vi "ASYNC_Adam_client.vi"(2 "Values":dbl[](array[numeric]) format="%.2f", 3 "Check Value is in the scan table?":bool, 4 "Channel Names":string[](array[string])) -> (0 "Scan Comments":string[](array[string]), 1 "Calibrated Units":dbl[](array[numeric]) format="%.4f")   [LabVIEW 2017]
uses:
  Anemometry/Anemometry Sub Vis/Controls/Global_mode.ctl
  Sub VIs/ADAM Controls/Update_scan_value.ctl
  Anemometry/Anemometry Sub Vis/Globals/Preference_global.vi
panel:
  out "Iterations":i32
  in  "ASYNC Adam server":refnum<vi>
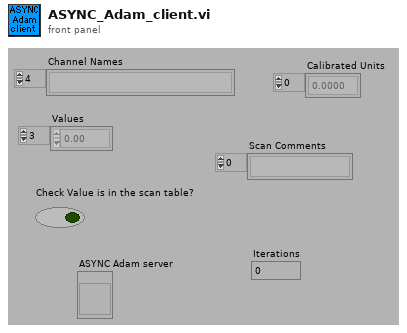
[diagram p1: front panel]
types:
  T1 = typedef "Server_Comms.ctl" = enum16{"Server Link Healthy", "Do Not Link To Server"}
  T2 = typedef "Update_scan_value.ctl" = cluster{"Channel Name":string, "New Value":dbl}
  T3 = typedef "Global_mode.ctl" = enum16{"Read Global", "Load Global From File", "Write Global to File"}
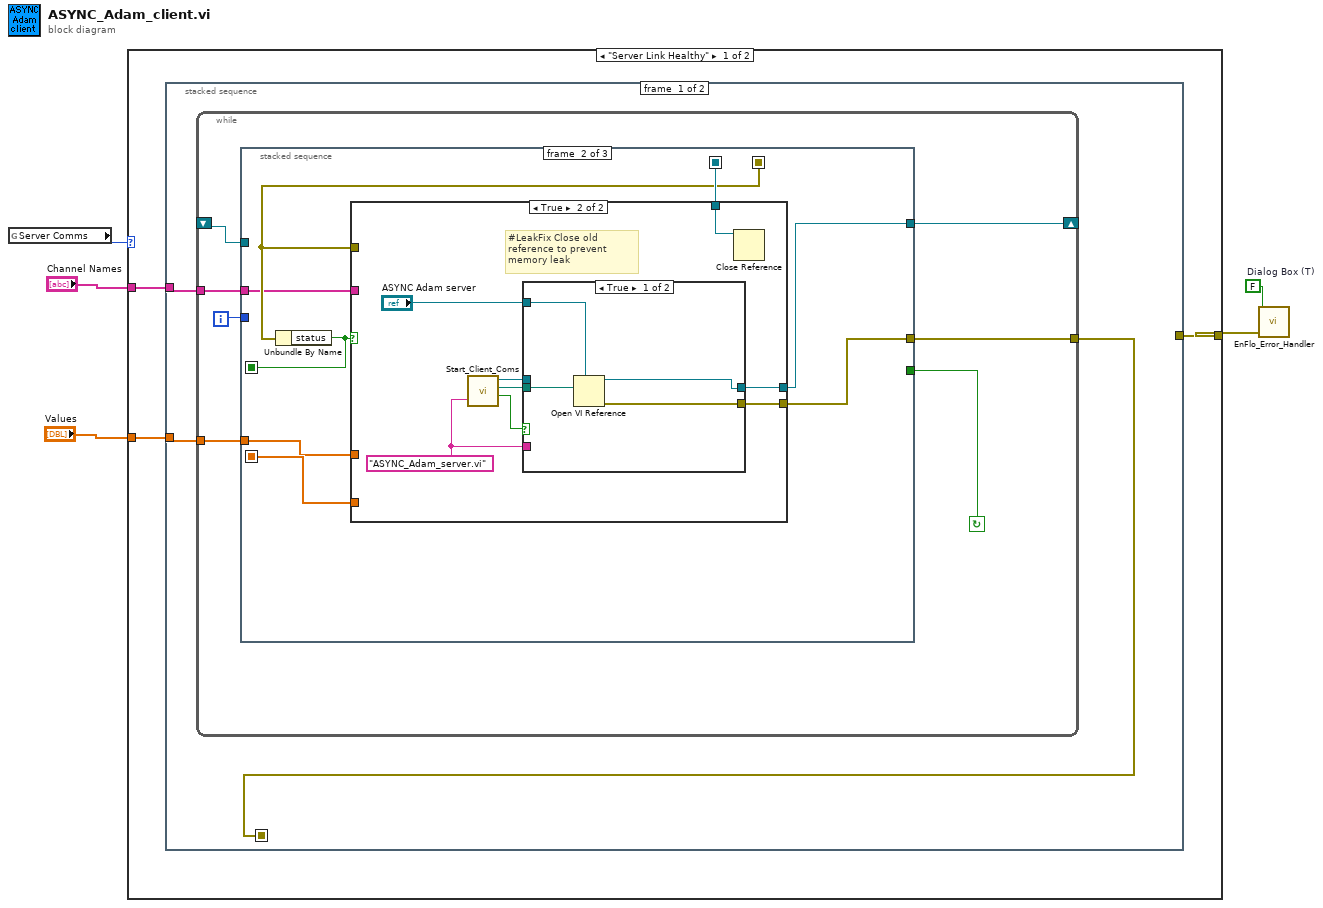
[diagram p0: block diagram]
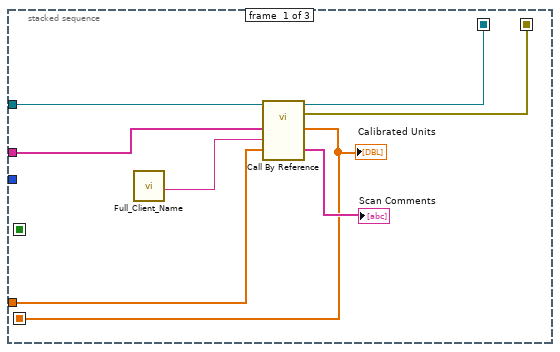
[diagram p2: hidden frame]
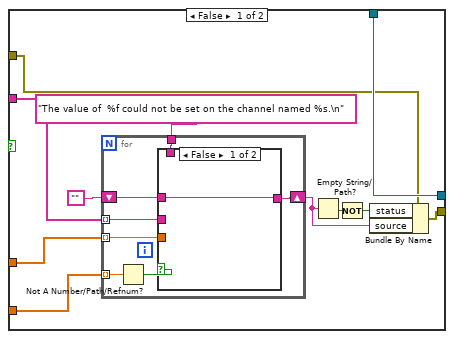
[diagram p3: hidden frame]
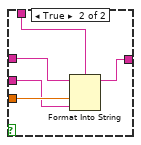
[diagram p4: hidden frame]
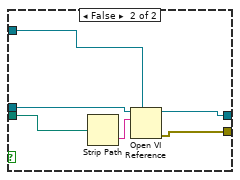
[diagram p5: hidden frame]
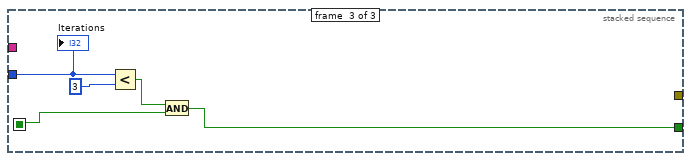
[diagram p6: hidden frame]
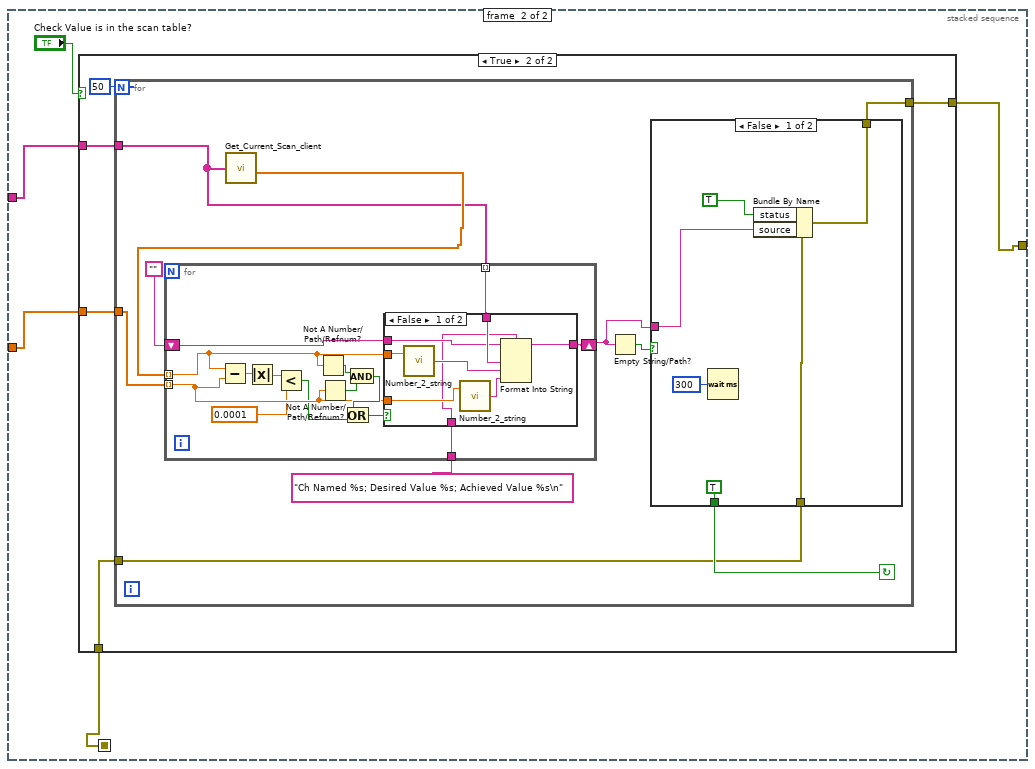
[diagram p7: hidden frame]
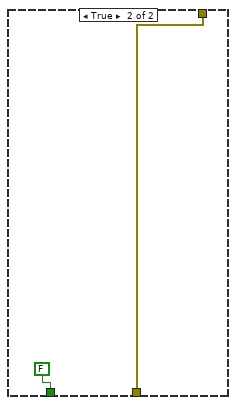
[diagram p10: hidden frame]
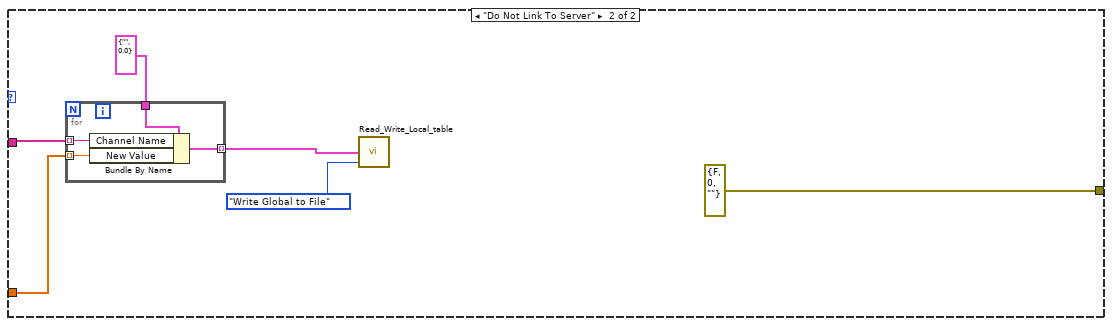
[diagram p11: hidden frame]
diagram:
  w1 = FALSE  # Dialog Box (T)
  n1 = global read "Preference_global.vi" "Server Comms"() -> (w4:T1)
  n2 = case shown="\"Server Link Healthy\"" w4 {
    tunnel: [w8 errorcluster {"status"=FALSE, "code"=0, "source"=""}] -> w5
    tunnel: "Channel Names" -> [w7 w136]
    tunnel: "Values" -> [w6 w135]
    frame "Server Link Healthy" {
      n3 = stacked-sequence {
        seq-local: [w9 _] -> [_ w83]
        tunnel: [_ w82] -> w8
        tunnel: w7 -> [w11 w85]
        tunnel: w6 -> [w10 w84]
        frame #0 {
          n4 = while {
            tunnel: w10 -> [w12]
            tunnel: w11 -> [w13]
            tunnel: [w14] -> w9
            shift-left: _ -> [w18]
            shift-right: [w17] -> _
            i -> [w16]
            stop <- w15 continue-if-true
            n5 = stacked-sequence {
              seq-local: [w24 _ _] -> [_ w34 _]
              seq-local: [w26 _ _] -> [_ w32 _]
              seq-local: [_ w33 _] -> [_ _ w78]
              seq-local: [w19 _ _] -> [_ w30 _]
              tunnel: w18 -> [w25 _ _]
              tunnel: [_ w31 _] -> w17
              tunnel: w16 -> [_ _ w79]
              tunnel: [_ _ w77] -> w15
              tunnel: [_ w27 _] -> w14
              tunnel: w13 -> [w22 w28 _]
              tunnel: w12 -> [w21 w29 _]
              frame #0 {
                n6 = call "Full_Client_Name.vi"() -> ("Client Name"=w20:string)
                n7 = call-by-ref "?"(reference=w25, "Values"=w21, "Client Name"=w20, "Channel Names"=w22) -> (reference out=w24:refnum<vi>, error out=w26:errorcluster, "Scan Comments"=→"Scan Comments":string[], "Calibrated Units"=w19:dbl[])  [unwired: 2 in]
                "Calibrated Units" <- w19
              }
              frame #1 {
                n8 = Unbundle By Name(w32) -> ("status"=w33:bool)
                n9 = case shown="True" w33 {
                  tunnel: w34 -> [w45 w59]
                  tunnel: [w38 w63] -> w27
                  tunnel: w32 -> [w39 _]
                  tunnel: [w45 w62] -> w31
                  tunnel: w30 -> [w44 _]
                  tunnel: w29 -> [w43 _]
                  tunnel: w28 -> [w42 _]
                  frame False {
                    n10 = for {
                      shift-right: [w47] -> w35
                      shift-left: "" -> [w48]
                      tunnel: w44 -> [w52] mode=indexing
                      tunnel: w43 -> [w50] mode=indexing
                      tunnel: w42 -> [w49] mode=indexing
                      tunnel: "The value of  %f could not be set on the channel named %s.\n" ("format string") -> [w46]
                      n11 = Not A Number/Path/Refnum?(number/path/refnum=w52) -> (NaN/Path/Refnum?=w51:bool)
                      n12 = case shown="False" w51 {
                        tunnel: w50 -> [_ w58]
                        tunnel: w49 -> [_ w57]
                        tunnel: w48 -> [w53 w56]
                        tunnel: [w53 w55] -> w47
                        tunnel: w46 -> [_ w54]
                        frame False {
                        }
                        frame True {
                          n13 = Format Into String(format string=w54, initial string=w56, w58, w57) -> (resulting string=w55:string)  [unwired: 1 in, 1 out]
                        }
                      }
                    }
                    n14 = Empty String/Path?(string/path=w35) -> (empty?=w37:bool)
                    n15 = Not(x=w37) -> (.not. x?=w36:bool)
                    n16 = Bundle By Name(cluster=w39, "status"=w36, "source"=w35) -> (w38:errorcluster)
                  }
                  frame True {
                    w61 = "ASYNC_Adam_server.vi"
                    # "#LeakFix Close old reference to prevent memory leak"
                    n17 = call "Start_Client_Coms.vi"("VI name to run on server"=w61) -> ("LabVIEW application reference"=w66:refnum<vi>, "Checked VI name"=w64:path, "Local Call"=w65:bool)  [unwired: 1 in, 1 out]
                    n18 = case shown="True" w65 {
                      tunnel: w64 -> [w70 w73]
                      tunnel: w66 -> [_ w71]
                      tunnel: [w69 w74] -> w63
                      tunnel: [w68 w75] -> w62
                      tunnel: w61 -> [_ _]
                      tunnel: "ASYNC Adam server" -> [w67 w72]
                      frame True {
                        n19 = Open VI Reference(type specifier VI Refnum (for type only)=w67, vi path=w70) -> (vi reference=w68:refnum<vi>, error out=w69:errorcluster)  [unwired: 1 in, 3 out]
                      }
                      frame False {
                        n20 = Strip Path(path=w73) -> (name=w76:string)  [unwired: 1 out]
                        n21 = Open VI Reference(type specifier VI Refnum (for type only)=w72, application reference (local)=w71, vi path=w76) -> (vi reference=w75:refnum<vi>, error out=w74:errorcluster)  [unwired: 1 in, 2 out]
                      }
                    }
                    n22 = Close Reference(reference=w59) -> ()  [unwired: 1 in, 1 out]
                  }
                }
              }
              frame #2 {
                n23 = Less?(x=w79, y=3) -> (x < y?=w81:bool)
                n24 = And(x=w81, y=w78) -> (x .and. y?=w77:bool)
                "Iterations" <- w79
              }
            }
          }
        }
        frame #1 {
          n25 = case shown="True" "Check Value is in the scan table?" {
            tunnel: w85 -> [_ w91]
            tunnel: w84 -> [_ w90]
            tunnel: w83 -> [w87 w89]
            tunnel: [w87 w88] -> w82
            frame False {
            }
            frame True {
              n26 = for {
                N: 50 -> [_]
                tunnel: w91 -> [w98]
                tunnel: w90 -> [w99]
                tunnel: [w94] -> w88
                tunnel: w89 -> [w93]
                stop <- w95 continue-if-true
                n27 = call "Get_Current_Scan_client.vi"("ADAM Ch Names"=w98) -> ("Numerical Values"=w100:dbl[])  [unwired: 3 out]
                n28 = for {
                  shift-right: [w115] -> w96
                  shift-left: "" -> [w114]
                  tunnel: w99 -> [w107] mode=indexing
                  tunnel: w100 -> [w108] mode=indexing
                  tunnel: "Ch Named %s; Desired Value %s; Achieved Value %s\n" ("format string") -> [w116]
                  tunnel: w98 -> [w109] mode=indexing
                  n29 = Subtract(x=w108, y=w107) -> (x-y=w106:dbl)
                  n30 = Absolute Value(x=w106) -> (abs(x)=w105:dbl)
                  n31 = Less?(x=w105, y=0.0001) -> (x < y?=w103:bool)
                  n32 = Not A Number/Path/Refnum?(number/path/refnum=w108) -> (NaN/Path/Refnum?=w111:bool)
                  n33 = Not A Number/Path/Refnum?(number/path/refnum=w107) -> (NaN/Path/Refnum?=w112:bool)
                  n34 = And(x=w111, y=w112) -> (x .and. y?=w110:bool)
                  n35 = Or(x=w110, y=w103) -> (x .or. y?=w113:bool)
                  n36 = case shown="False" w113 {
                    tunnel: w109 -> [w124 _]
                    tunnel: w108 -> [w118 _]
                    tunnel: w107 -> [w119 _]
                    tunnel: w116 -> [w117 _]
                    tunnel: [w123 w125] -> w115
                    tunnel: w114 -> [w122 w125]
                    frame False {
                      n37 = call "Number_2_string.vi"("number"=w118) -> ("String"=w120:string)  [unwired: 1 in]
                      n38 = call "Number_2_string.vi"("number"=w119) -> ("String"=w121:string)  [unwired: 1 in]
                      n39 = Format Into String(format string=w117, initial string=w122, w124, w120, w121) -> (resulting string=w123:string)  [unwired: 1 in, 1 out]
                    }
                    frame True {
                    }
                  }
                }
                n40 = Empty String/Path?(string/path=w96) -> (empty?=w97:bool)
                n41 = case shown="False" w97 {
                  tunnel: [TRUE FALSE] -> w95
                  tunnel: w96 -> [w131 _]
                  tunnel: [w130 w132] -> w94
                  tunnel: w93 -> [w129 w132]
                  frame False {
                    n42 = Wait (ms)(milliseconds to wait=u32 300) -> ()  [unwired: 1 out]
                    n43 = Bundle By Name(cluster=w129, "status"=TRUE, "source"=w131) -> (w130:errorcluster)
                  }
                  frame True {
                  }
                }
              }
            }
          }
        }
      }
    }
    frame "Do Not Link To Server" {
      n44 = for {
        tunnel: T2 {"Channel Name"="", "New Value"=0.0} ("Update Scan Value Cluster") -> [w143]
        tunnel: w136 -> [w142] mode=indexing
        tunnel: w135 -> [w141] mode=indexing
        tunnel: [w140] -> w134 mode=indexing
        n45 = Bundle By Name(cluster=w143, "Channel Name"=w142, "New Value"=w141) -> (w140:T2)
      }
      n46 = call "Read_Write_Local_table.vi"("Mode"=Global_mode."Write Global to File", "Ch Values in"=w134) -> ()  [unwired: 1 in, 3 out]
    }
  }
  n47 = call "EnFlo_Error_Handler.vi"("error in (no error)"=w5, "Dialog Box (T)"=w1) -> ()  [unwired: 1 in, 3 out]
